vi "Global GUI indicator ref cluster.vi"() -> ()   [LabVIEW 2014]
uses:
  GUI indicator reference cluster.ctl
panel:
  out "GUI indicator cluster reference":T1
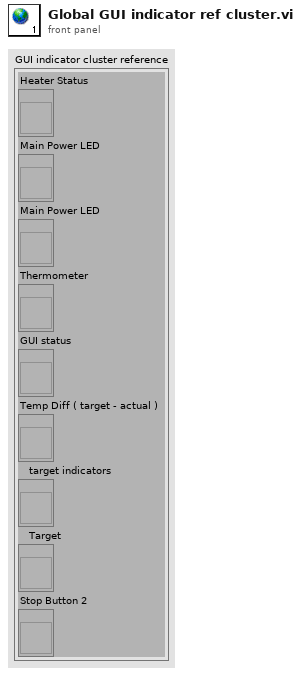
[diagram p1: front panel]
types:
  T1 = typedef "GUI indicator reference cluster.ctl" = cluster{"Heater Status":refnum<vi>, "Main Power LED":refnum<vi>, "Main Power LED":refnum<vi>, "Thermometer":refnum<vi>, "GUI status":refnum<vi>, "Temp Diff ( target - actual )":refnum<vi>, "   target indicators":refnum<vi>, "   Target":refnum<vi>, "Stop Button 2":refnum<vi>}
diagram:
